vi "Device Class Selection.vi"(4 "Device Class Strings":string[](array[string]), 5 "Device Classes":T1) -> (1 "Device Class":string[](array[string]))   [LabVIEW 2015, in "SMI.lvlib" / "Device.lvclass"]
uses:
  Device.lvclass
  Controls/DeviceClassSelection.ctl
panel:
  out "error out":errorcluster
  in  "error in":errorcluster
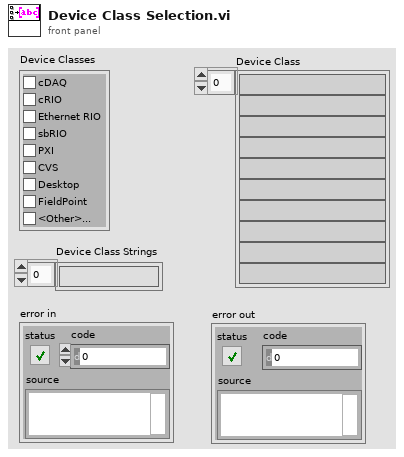
[diagram p1: front panel]
types:
  T1 = typedef "SMI.lvlib/Device.lvclass/DeviceClassSelection.ctl" = cluster{"cDAQ":bool, "cRIO":bool, "Ethernet RIO":bool, "sbRIO":bool, "PXI":bool, "CVS":bool, "Desktop":bool, "FieldPoint":bool, "<Other>...":bool}
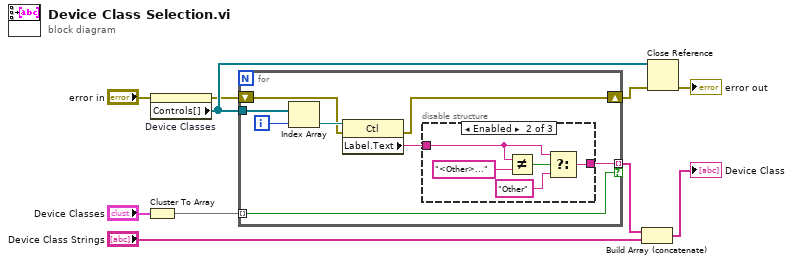
[diagram p0: block diagram]
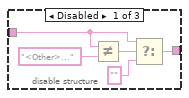
[diagram p2: hidden frame]
diagram:
  n1 = Cluster To Array(cluster="Device Classes") -> (array=w9:bool[])
  n2 = property on="Device Classes" class="Clust (strict)"(error in="error in") -> (error out=w7:errorcluster, "Controls[]"=w8:refnum<vi>[])  [unwired: 1 in, 1 out]
  n3 = for {
    tunnel: w9 -> [w18] mode=indexing
    tunnel: [w11] -> w3 mode=indexing if=w18
    tunnel: w8 -> [w15]
    shift-right: [w13] -> w5
    shift-left: w7 -> [w14]
    i -> [w17]
    n4 = Index Array(array=w15, index=w17) -> (element=w16:refnum<vi>)
    n5 = property class="Ctl"(reference=w16, error in=w14) -> (error out=w13:errorcluster, "Label.Text"=w12:string)  [unwired: 1 out]
    n6 = disable-structure shown="Enabled" {
      disable-tunnel: w12 -> [w21 w26 w29]
      disable-tunnel: [w19 w24 w29] -> w11
      frame Disabled {
        n7 = Not Equal?(x=w21, y="<Other>...") -> (x != y?=w22:bool)
        n8 = Select(t=w21, s=w22, f="") -> (s? t:f=w19:string)
      }
      frame Enabled {
        n9 = Not Equal?(x=w26, y="<Other>...") -> (x != y?=w27:bool)
        n10 = Select(t=w26, s=w27, f="Other") -> (s? t:f=w24:string)
      }
      frame Disabled {
      }
    }
  }
  n11 = Build Array (concatenate)(w3, "Device Class Strings") -> (→"Device Class":string[])
  n12 = Close Reference(reference=w8, error in (no error)=w5) -> (error out=→"error out":errorcluster)
